vi "IP Address Finder.vi"() -> ()   [LabVIEW 2017]
panel:
  in  "stop":bool
  out "size(s)":i32
  out "All Other IP Addresses":string
  out "Primary IP Address":string
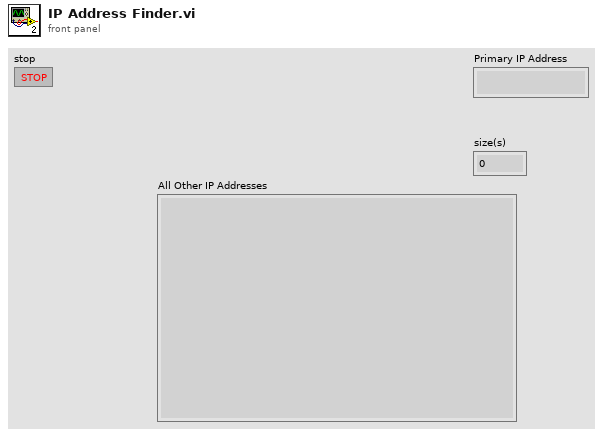
[diagram p1: front panel]
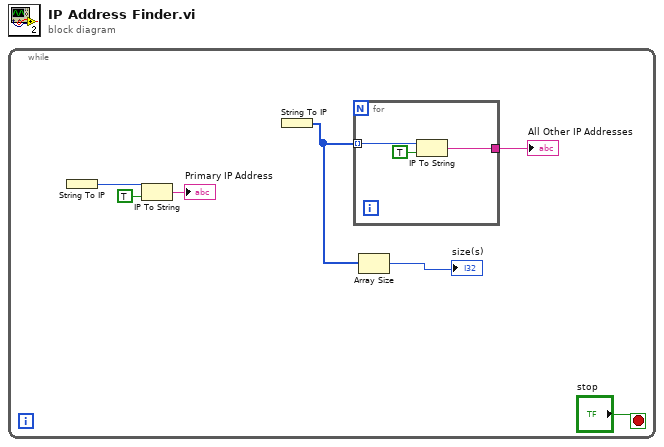
[diagram p0: block diagram]
diagram:
  n1 = while {
    stop <- "stop" stop-if-true
    n2 = String To IP() -> (0:w7:u32)  [unwired: 1 in]
    n3 = IP To String(1:TRUE ("dot notation? (F)"), 2:w7) -> (0:→"Primary IP Address":string)
    n4 = String To IP() -> (0:w3:u32[])  [unwired: 1 in]
    n5 = for {
      tunnel: w3 -> [w10] mode=indexing
      tunnel: [w8] -> w4
      n6 = IP To String(1:TRUE ("dot notation? (F)"), 2:w10) -> (0:w8:string)
    }
    "All Other IP Addresses" <- w4
    n7 = Array Size(array=w3) -> (size(s)=→"size(s)":i32)
  }
